vi "TrancateData(SubVI).vi"(9 "TotalLength(200)":i32=300, 10 "prePeakPoints(40)":i32=150, 11 "DataIn":dbl[](array[numeric])) -> (3 "DataOut":dbl[](array[numeric]))   [LabVIEW 2024]
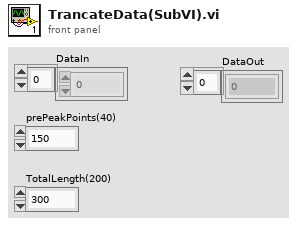
[diagram p1: front panel]
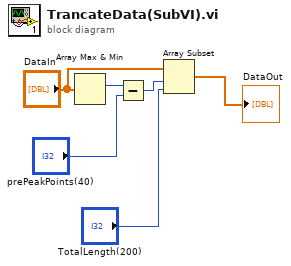
[diagram p0: block diagram]
diagram:
  n1 = Array Max & Min(array="DataIn") -> (max index (indices)=w5:i32)  [unwired: 3 out]
  n2 = Subtract(x=w5, y="prePeakPoints(40)") -> (x-y=w6:i32)
  n3 = Array Subset(array="DataIn", index=w6, length="TotalLength(200)") -> (→"DataOut":dbl[])
